vi "Write Current_Share.vi"(8 "error in":errorcluster, 10 "Current_Sharing":bool, 11 "69X_79X in":refnum<class "6972A.lvclass">) -> (0 "error out":errorcluster, 3 "69X_79X out":refnum<class "6972A.lvclass">)   [LabVIEW 2019, in "6972A.lvlib" / "6972A.lvclass"]
uses:
  Library/6972A.lvclass
  builds/Instruments/PowerSupply.lvlibp/Library/PowerSupply.lvclass
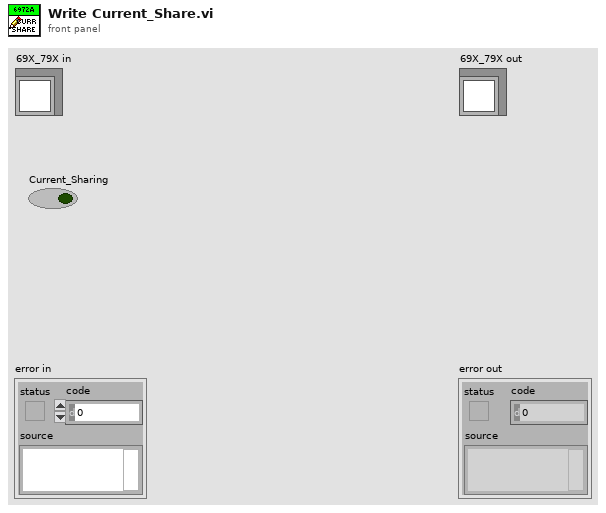
[diagram p1: front panel]
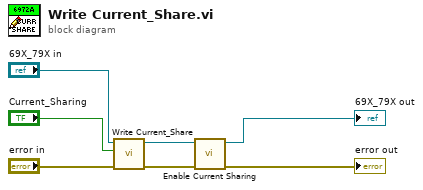
[diagram p0: block diagram]
diagram:
  n1 = call-parent "Write Current_Share.vi"("error in"="error in", "Current_Sharing"="Current_Sharing", "PowerSupply in"="69X_79X in") -> ("error out"=w3:errorcluster, "PowerSupply out"=w4:refnum<class "6972A.lvclass">)  [unwired: 7 in]
  n2 = call "Enable Current Sharing.vi"("error in (no error)"=w3, "69X_79X in"=w4) -> ("error out"=→"error out":errorcluster, "69X_79X out"=→"69X_79X out":refnum<class "6972A.lvclass">)  [unwired: 8 in]
